vi "FPGA.vi"() -> ()   [LabVIEW 2018]
uses:
  <vilib>/rvi/Emulation/niFpgaGetClockAttributes.vi
  <vilib>/rvi/Emulation/niFpgaSctlEmulationGetInTimedLoop.vi
  <vilib>/rvi/Emulation/niFpgaEmulationReportErrorSimple.vi
  <vilib>/rvi/eio/common/nirviEmuTemplateMethod_errors.vi
  <vilib>/rvi/interface/RandomDataEmulation/niFpgaRandomDataHandleErrors.vi
  <vilib>/rvi/Emulation/niFpgaCriticalErrorInLSC.vi
  <vilib>/eio/EIONode/EIONode.xnode
  <vilib>/rvi/DataTransferAndStorage/Container/XNode/niFpgaContainer.xnode
  <vilib>/rvi/interface/RandomDataEmulation/nirviRandomDataFpgaReadWriteTemplate.vi
panel:
  out "Waveform Chart 2":i16(graph)
  out "Waveform Chart":i16(graph)
  out "Timed Out?":bool
  out "x-y":u32
  in  "stop":bool
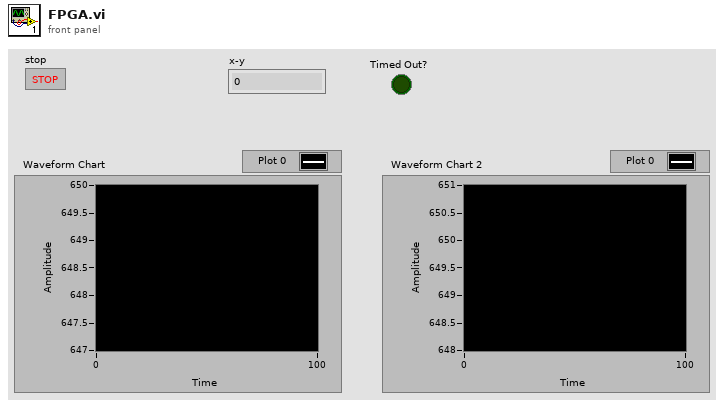
[diagram p1: front panel]
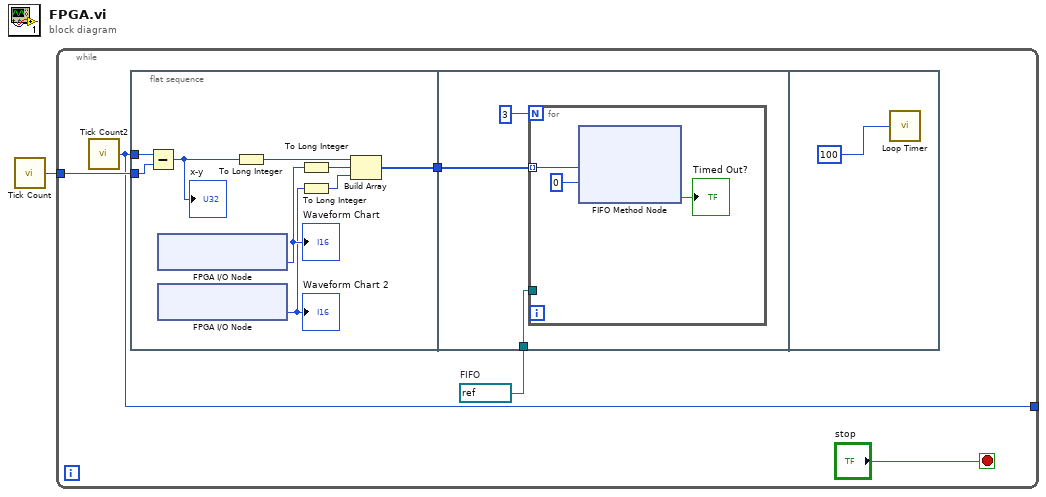
[diagram p0: block diagram]
diagram:
  n1 = call "Tick Count"() -> ("Tick Count(uSec)"=w1:u32)
  n2 = while {
    tunnel: w1 -> [w6]
    tunnel: [w4] -> _
    stop <- "stop" stop-if-true
    w2 = refnum<k21> "FIFO"  # FIFO
    n3 = call "Tick Count2"() -> ("Tick Count(uSec)"=w4:u32)
    n4 = flat-sequence {
      tunnel: w6 -> [w15]
      tunnel: w4 -> [w14]
      tunnel: [w13] -> w3
      tunnel: w3 -> [w18]
      tunnel: w2 -> [w16]
      frame #0 {
        n5 = Subtract(x=w14, y=w15) -> (x-y=w12:u32)
        "x-y" <- w12
        n6 = xnode "FPGA I/O Node"() -> ("ConnectorC/AI0"=w9:i16)  [unwired: 1 in, 1 out]
        "Waveform Chart" <- w9
        n7 = xnode "FPGA I/O Node"() -> ("ConnectorC/AI1"=w7:i16)  [unwired: 1 in, 1 out]
        "Waveform Chart 2" <- w7
        n8 = To Long Integer(number=w12) -> (32bit integer=w11:i32)
        n9 = To Long Integer(number=w9) -> (32bit integer=w10:i32)
        n10 = To Long Integer(number=w7) -> (32bit integer=w8:i32)
        n11 = Build Array(w11, w10, w8) -> (w13:i32[])
      }
      frame #1 {
        n12 = for {
          N: 3 -> [_]
          tunnel: w18 -> [w20] mode=indexing
          tunnel: w16 -> [_]
          n13 = xnode ("FIFO Method Node")("Element"=w20, "Timeout"=0) -> ("Timed Out?"=→"Timed Out?":bool)  [unwired: 1 in, 1 out]
        }
      }
      frame #2 {
        n14 = call "Loop Timer"("Count(uSec)"=u32 100) -> ()  [unwired: 1 out]
      }
    }
  }
